vi "niFPGA Convert LUT Val to Hanning U16.vi"(0 "LUT value":u32, 9 "fractional index":u16) -> (6 "Hanning (U16)":u16)   [LabVIEW 2017]
uses:
  <vilib>/rvi/Arithmetic/AddSubMult/XNode/nirviSatArithmetic.xnode
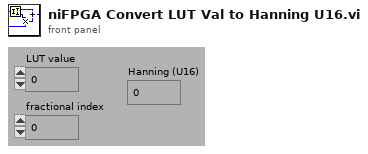
[diagram p1: front panel]
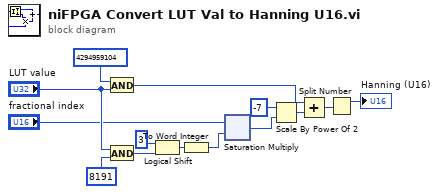
[diagram p0: block diagram]
diagram:
  n1 = And(x=u32 4294959104, y="LUT value") -> (x .and. y?=w13:u32)
  n2 = And(x="LUT value", y=u32 8191) -> (x .and. y?=w11:u32)
  n3 = Logical Shift(y=i8 3 ("n"), x=w11) -> (x << y=w12:u32)
  n4 = To Word Integer(number=w12) -> (16bit integer=w2:i16)
  n5 = xnode "Saturation Multiply"("x"="fractional index", "y"=w2) -> ("x*y"=w1:i32)
  n6 = Scale By Power Of 2(n=i8 -7, x=w1) -> (x*2^n=w10:i32)
  n7 = Add(x=w13, y=w10) -> (x+y=w6:u32)
  n8 = Split Number(x=w6) -> (hi(x)=→"Hanning (U16)":u16)  [unwired: 1 out]
